vi "Construct.vi"(11 "Serial Configuration":T1) -> (3 "MelsecMcNet out":refnum<class "MelsecFxLinks.lvclass">)   [LabVIEW 2020, in "MelsecFxLinks.lvclass"]
uses:
  MelsecFxLinks.lvclass
  MelsecFxLinks.lvclass/MelsecFxLinks.ctl
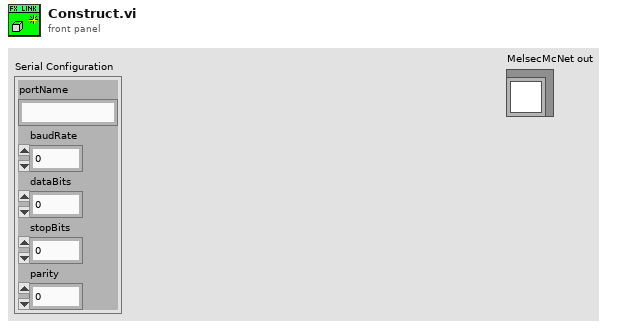
[diagram p1: front panel]
types:
  T1 = cluster{"portName":string, "baudRate":i32, "dataBits":i32, "stopBits":i32, "parity":i32}
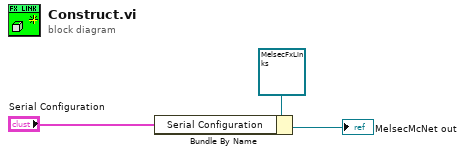
[diagram p0: block diagram]
diagram:
  n1 = Bundle By Name(cluster=refnum<class "MelsecFxLinks.lvclass"> refnum ("MelsecMcNet in"), "Serial Configuration"="Serial Configuration") -> (→"MelsecMcNet out":refnum<class "MelsecFxLinks.lvclass">)
